vi "Arrange Controls.vi"(0 "VI in":refnum<vi>, 5 "front panel":refnum<vi>, 11 "error in":errorcluster) -> (4 "VI out":refnum<vi>, 15 "error out":errorcluster)   [LabVIEW 2014]
uses:
  <vilib>/Utility/miscctls.llb/LVRectTypeDef.ctl
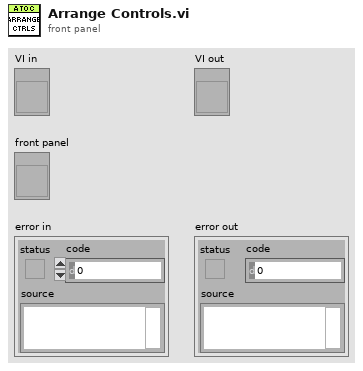
[diagram p1: front panel]
types:
  T1 = enum32{"invalid VI type", "Standard VI", "Control VI", "Global VI", "Polymorphic VI", "Configuration VI", "SubSystem", "Facade VI", "Method VI", "Statechart Diagram VI"}
  T2 = typedef "LVRectTypeDef.ctl" = cluster{"Left":i16, "Top":i16, "Right":i16, "Bottom":i16}
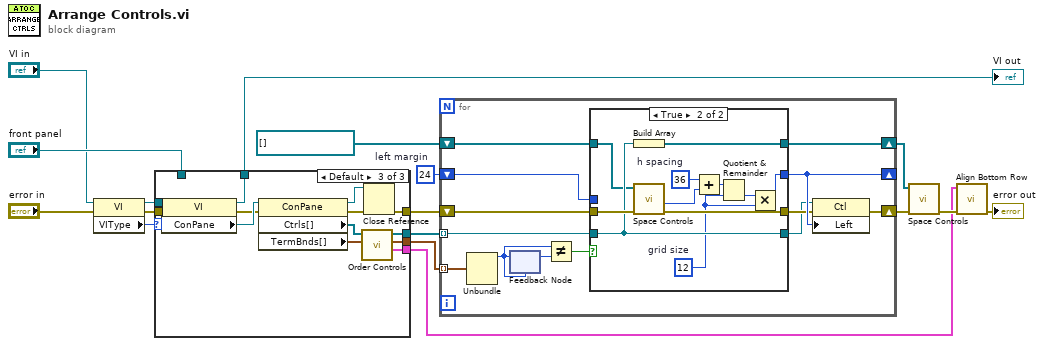
[diagram p0: block diagram]
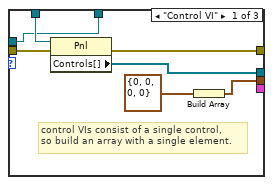
[diagram p2: hidden frame]
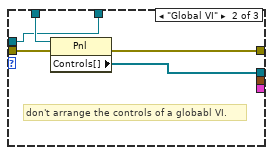
[diagram p3: hidden frame]
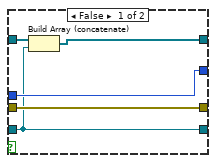
[diagram p4: hidden frame]
diagram:
  w4 = 24  # left margin
  n1 = property class="VI"(reference="VI in", error in="error in") -> (reference out=w13:refnum<vi>, error out=w15:errorcluster, "VIType"=w16:T1)
  n2 = case shown="Default" w16 {
    tunnel: [w21 _ w38] -> w8
    tunnel: [w23 w28 w37] -> w9
    tunnel: [w20 w27 w34] -> w10
    tunnel: [_ _ w33] -> w1
    tunnel: [w18 w25 w32] -> w11
    tunnel: w13 -> [w18 w25 w31]
    tunnel: w15 -> [w19 w26 w30]
    tunnel: "front panel" -> [w24 w29 _]
    frame "Control VI" {
      # "control VIs consist of a single control,\nso build an array with a single element."
      n3 = property class="Pnl"(reference=w24, error in=w19) -> (error out=w20:errorcluster, "Controls[]"=w23:refnum<vi>[])  [unwired: 1 out]
      n4 = Build Array(T2 {"Left"=0, "Top"=0, "Right"=0, "Bottom"=0} ("Rectangle")) -> (w21:T2[])
    }
    frame "Global VI" {
      # "don't arrange the controls of a globabl VI."
      n5 = property class="Pnl"(reference=w29, error in=w26) -> (error out=w27:errorcluster, "Controls[]"=w28:refnum<vi>[])  [unwired: 1 out]
    }
    frame Default {
      n6 = property class="VI"(reference=w31, error in=w30) -> (reference out=w32:refnum<vi>, error out=w39:errorcluster, "ConPane"=w40:refnum<vi>)
      n7 = property class="ConPane"(reference=w40, error in=w39) -> (reference out=w35:refnum<vi>, error out=w36:errorcluster, "Ctrls[]"=w42:refnum<vi>[], "TermBnds[]"=w41:T2[])
      n8 = call "Order Controls.vi"("TermBnds[]"=w41, "Controls in"=w42) -> ("sorted array"=w33:cluster{"Rectangle":T2, refnum<vi>}[], "Control locations"=w38:T2[], "Controls out"=w37:refnum<vi>[])  [unwired: 7 in]
      n9 = Close Reference(reference=w35, error in (no error)=w36) -> (error out=w34:errorcluster)
    }
  }
  "VI out" <- w11
  n10 = for {
    shift-right: [w54] -> w7
    shift-left: refnum<vi>[] [] -> [w53]
    shift-right: [w50] -> _
    shift-left: w4 -> [w51]
    tunnel: w9 -> [w46] mode=indexing
    shift-right: [w48] -> w6
    shift-left: w10 -> [w47]
    tunnel: w8 -> [w44] mode=indexing
    n11 = Unbundle(w44) -> ("Left"=w43:i16)  [unwired: 3 out]
    n12 = feedback-in #1(w43) -> ()
    n13 = feedback #1(w43) -> (w55:i16)
    n14 = Not Equal?(x=w43, y=w55) -> (x != y?=w52:bool)
    n15 = case shown="True" w52 {
      tunnel: [w60 w71] -> w54
      tunnel: w53 -> [w59 w65]
      tunnel: [w58 w61] -> w50
      tunnel: w51 -> [w58 _]
      tunnel: [w57 w70] -> w49
      tunnel: w47 -> [w57 w69]
      tunnel: w46 -> [w56 w68]
      tunnel: [w56 w68] -> w45
      frame False {
        n16 = Build Array (concatenate)(w59, w56) -> (w60:refnum<vi>[])
      }
      frame True {
        w63 = 12  # grid size
        w67 = 36  # h spacing
        n17 = Build Array(w68) -> (w71:refnum<vi>[])
        n18 = call "Space Controls.vi"("error in"=w69, "Controls in"=w65) -> ("error out"=w70:errorcluster, "Max right location"=w66:i32)  [unwired: 7 in, 1 out]
        n19 = Add(x=w67, y=w66) -> (x+y=w62:i32)
        n20 = Quotient & Remainder(x=w62, y=w63) -> (floor(x/y)=w64:i32)  [unwired: 1 out]
        n21 = Multiply(x=w64, y=w63) -> (x*y=w61:i32)
      }
    }
    n22 = property class="Ctl"(reference=w45, error in=w49, "Left"=w50) -> (error out=w48:errorcluster)  [unwired: 1 out]
  }
  n23 = call "Space Controls.vi"("error in"=w6, "Controls in"=w7) -> ("error out"=w3:errorcluster)  [unwired: 7 in, 2 out]
  n24 = call "Align Bottom Row.vi"("error in"=w3, "sorted array"=w1) -> ("error out"=→"error out":errorcluster)  [unwired: 9 in]
